vi "Write Instr Addr.vi"(8 "error in (no error)":errorcluster, 10 "Instr Addr":refnum<visa-resource-name>, 11 "Power Supply Parent in":refnum<class "Power Supply Parent.lvclass">) -> (0 "error out":errorcluster, 3 "Power Supply Parent out":refnum<class "Power Supply Parent.lvclass">)   [LabVIEW 2017, in "Power Supply Driver.lvlib" / "Power Supply Parent.lvclass"]
uses:
  Power Supply Parent.lvclass
  Power Supply Parent.lvclass/Power Supply Parent.ctl
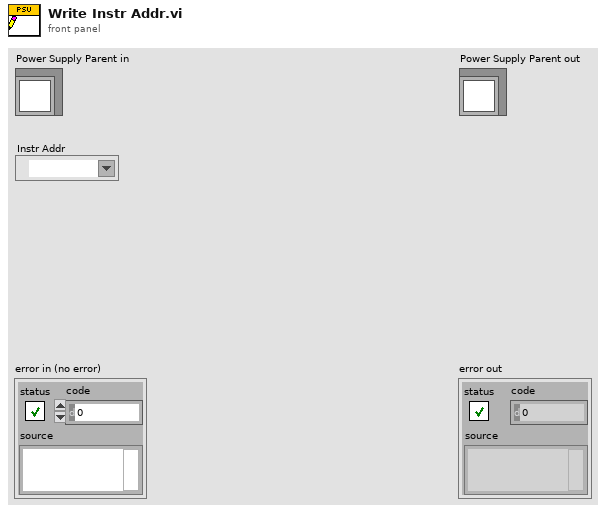
[diagram p1: front panel]
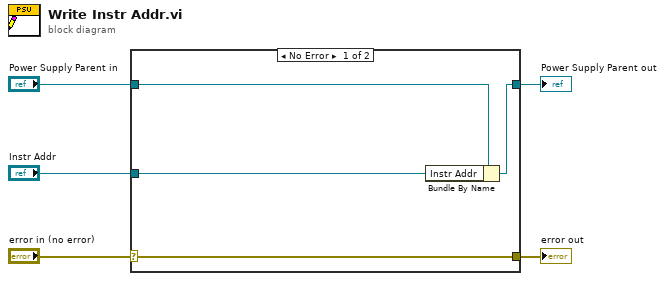
[diagram p0: block diagram]
diagram:
  n1 = case shown="No Error" "error in (no error)" {
    selector: "error in (no error)" -> [w9 w10]
    tunnel: [w9 w10] -> w4
    tunnel: [w7 w11] -> w2
    tunnel: "Power Supply Parent in" -> [w8 w11]
    tunnel: "Instr Addr" -> [w6 _]
    frame No Error {
      n2 = Bundle By Name(cluster=w8, "Instr Addr"=w6) -> (w7:refnum<class "Power Supply Parent.lvclass">)
    }
    frame Error {
    }
  }
  "error out" <- w4
  "Power Supply Parent out" <- w2
